vi "TreeItem.Get.vi"(6 "Custom Device Path":string, 8 "error in (no error)":errorcluster, 9 "Tree":T1[](array[typedef]) {"Properties"."Type" items=["K_STRING", "K_BOOL", "K_I32", "K_U32", "K_DOUBLE", "K_U64", "K_VARIANT", "K_DEPENDENTFILE", "K_DEPENDENTNODE", "K_DATASOURCENODE", "K_U16", "K_DBLARR", "K_U32ARR", "K_I32ARR", "K_STRINGARR", "K_DICTIONARY", "K_DICTIONARYARR"]}, 10 "BaseNode Ref":refnum<k24>, 11 "NodeIDUtil Ref":refnum<k24>) -> (0 "error out":errorcluster, 1 "Tree":T1[](array[typedef]) {"Properties"."Type" items=["K_STRING", "K_BOOL", "K_I32", "K_U32", "K_DOUBLE", "K_U64", "K_VARIANT", "K_DEPENDENTFILE", "K_DEPENDENTNODE", "K_DATASOURCENODE", "K_U16", "K_DBLARR", "K_U32ARR", "K_I32ARR", "K_STRINGARR", "K_DICTIONARY", "K_DICTIONARYARR"]}, 2 "BaseNode Ref out":refnum<k24>, 3 "NodeIDUtil Ref out":refnum<k24>)   [LabVIEW 2016, in "Advanced System Definition.lvlib"]
uses:
  SysDef API/Advanced System Definition.lvlib
  _Types/TreeItem.ctl
  _Types/TreeItem.Info.ctl
  <vilib>/NI Veristand/Custom Device API/Custom Device Channel.ctl
  <vilib>/NI Veristand/Custom Device API/Custom Device Channel Type.ctl
  <vilib>/NI Veristand/Custom Device API/Custom Device Waveform.ctl
  <vilib>/NI Veristand/Custom Device API/Custom Device Waveform DataType.ctl
  _Types/TreeItem.Property.ctl
  NationalInstruments.VeriStand.SystemStorage
  NationalInstruments.VeriStand.SystemDefinitionAPI
  <vilib>/NI VeriStand/Custom Device API/Custom Device API.lvlib
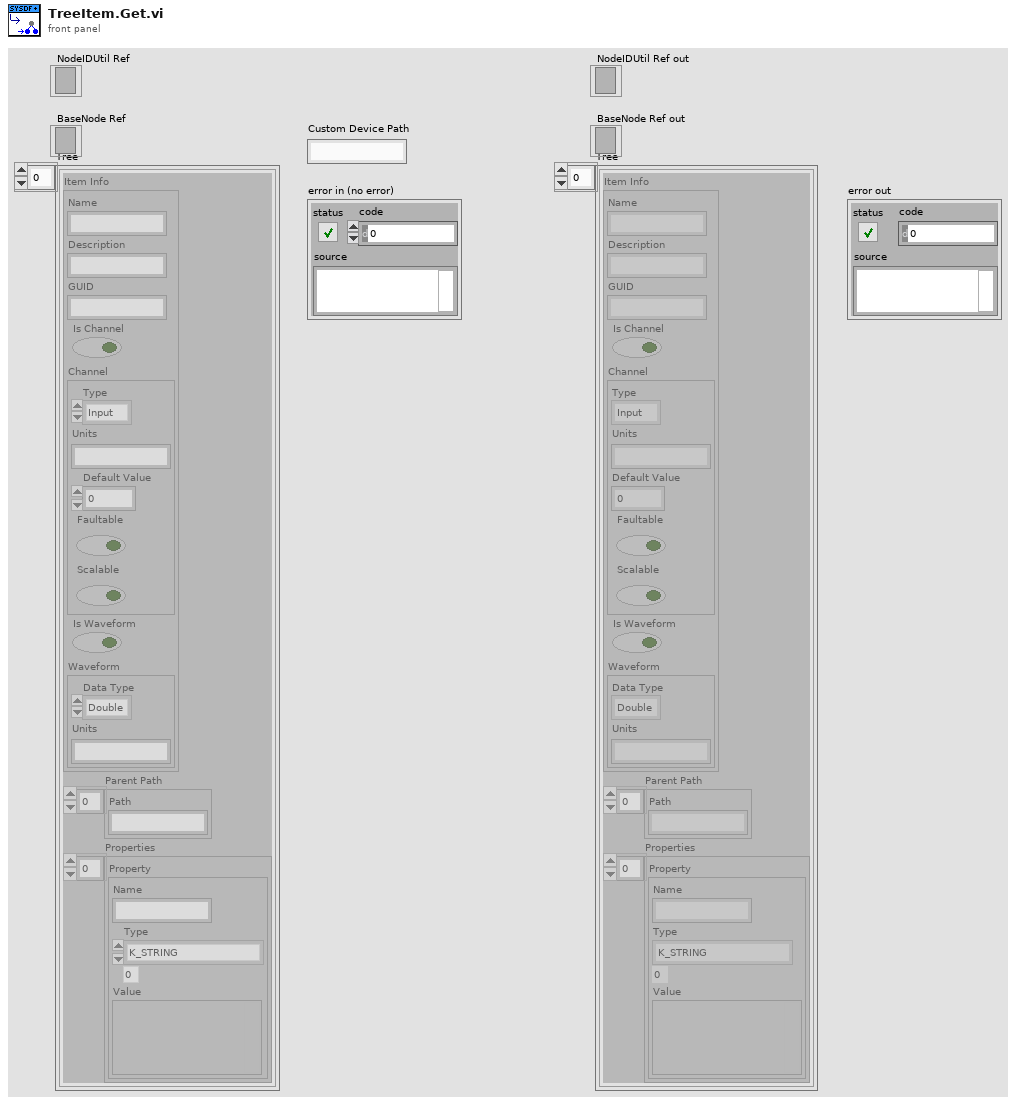
[diagram p1: front panel]
types:
  T1 = typedef "Advanced System Definition.lvlib/TreeItem.ctl" = cluster{"Item Info":T2, "Parent Path":string[], "Properties":T7[]}
  T2 = typedef "Advanced System Definition.lvlib/TreeItem.Info.ctl" = cluster{"Name":string, "Description":string, "GUID":string, "Is Channel":bool, "Channel":T3, "Is Waveform":bool, "Waveform":T5}
  T3 = typedef "Custom Device API.lvlib/Custom Device Channel.ctl" = cluster{"Type":T4, "Units":string, "Default Value":dbl, "Faultable":bool, "Scalable":bool}
  T4 = typedef "Custom Device API.lvlib/Custom Device Channel Type.ctl" = enum16{"Input", "Output"}
  T5 = typedef "Custom Device API.lvlib/Custom Device Waveform.ctl" = cluster{"Data Type":T6, "Units":string}
  T6 = typedef "Custom Device API.lvlib/Custom Device Waveform DataType.ctl" = enum16{"Double", "Complex Double"}
  T7 = typedef "Advanced System Definition.lvlib/TreeItem.Property.ctl" = cluster{"Name":string, "Type":i32, "Value":variant}
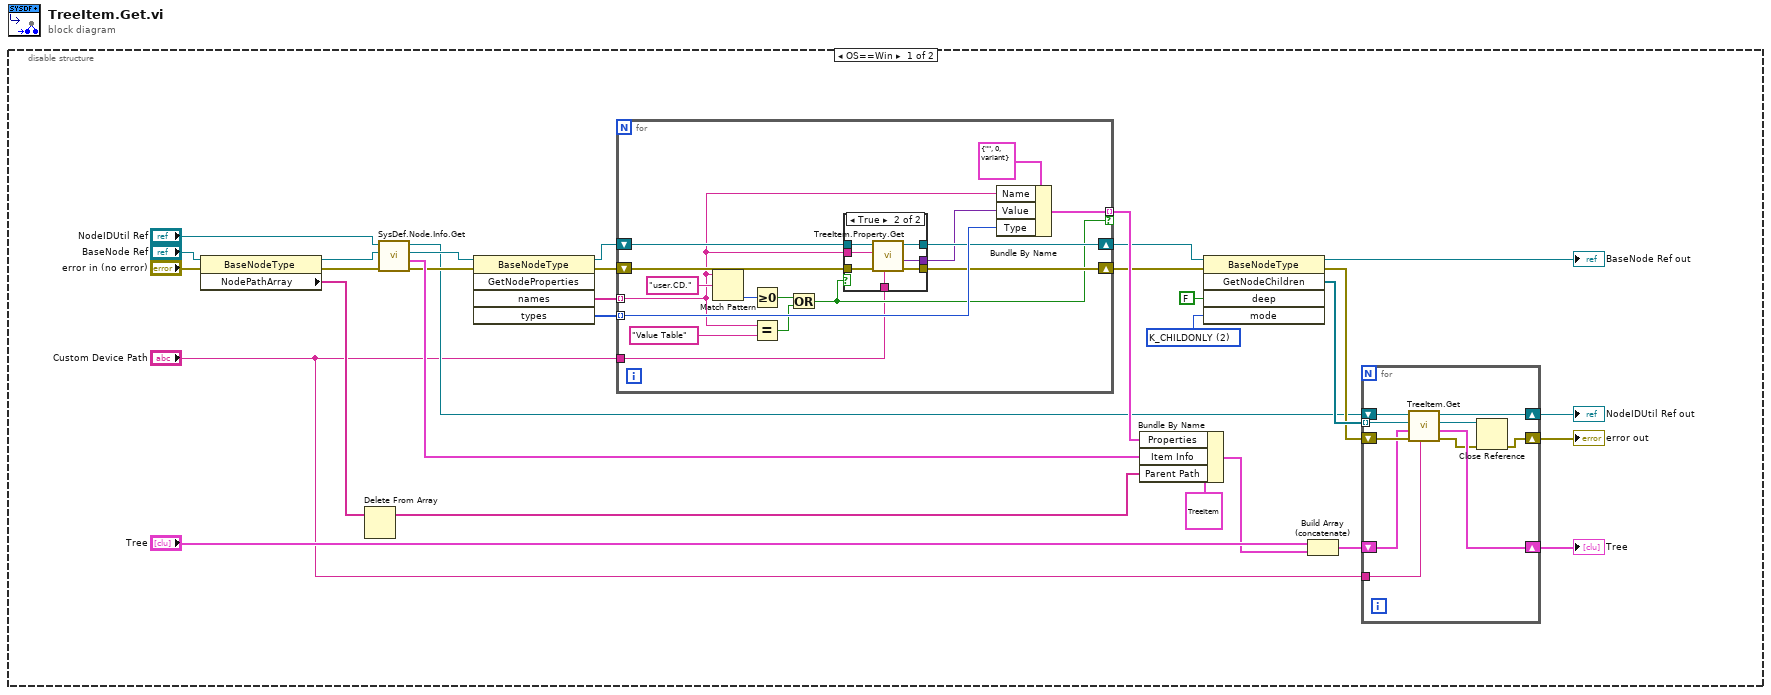
[diagram p0: block diagram]
diagram:
  n1 = disable-structure shown="OS==Win" {
    frame condition #0 (active) {
      w18 = 2 items=["K_BFS", "K_DFS", "K_CHILDONLY", "K_UP"] ("mode")
      n2 = property class="BaseNodeType"(reference="BaseNode Ref", error in="error in (no error)") -> (reference out=w6:refnum<k24>, error out=w9:errorcluster, "NodePathArray"=w7:string[])
      n3 = Delete From Array(array=w7) -> (array with subset deleted=w12:string[])  [unwired: 2 in, 1 out]
      n4 = call "SysDef.Node.Info.Get.vi"("error in (no error)"=w9, "BaseNode Ref"=w6, "NodeIDUtil Ref in"="NodeIDUtil Ref") -> ("error out"=w14:errorcluster, "Item Info"=w23:T2, "BaseNode Ref out"=w5:refnum<k24>, "NodeIDUtil Ref out"=w4:refnum<k24>)  [unwired: 5 in]
      n5 = invoke class="BaseNodeType" method="GetNodeProperties"(reference=w5, error in=w14) -> (reference out=w25:refnum<k24>, error out=w26:errorcluster, "names"=w28:string[], "types"=w27:i32[])  [unwired: 3 in, 1 out]
      n6 = for {
        tunnel: w27 -> [w52] mode=indexing
        tunnel: w28 -> [w47] mode=indexing
        shift-right: [w48] -> w21
        shift-left: w26 -> [w55]
        tunnel: [w51] -> w22 mode=indexing if=w43
        shift-right: [w50] -> w20
        shift-left: w25 -> [w54]
        tunnel: "Custom Device Path" -> [w42]
        n7 = Match Pattern(string=w47, regular expression="user.CD.") -> (offset past match=w56:i32)  [unwired: 1 in, 3 out]
        n8 = Greater Or Equal To 0?(x=w56) -> (x >= 0?=w44:bool)
        n9 = Equal?(x=w47, y="Value Table") -> (x = y?=w45:bool)
        n10 = Or(x=w44, y=w45) -> (x .or. y?=w43:bool)
        n11 = case shown="True" w43 {
          tunnel: w55 -> [w59 w66]
          tunnel: [w59 w65] -> w48
          tunnel: [_ w64] -> w49
          tunnel: w54 -> [w58 w63]
          tunnel: w47 -> [_ w62]
          tunnel: [w58 w61] -> w50
          tunnel: w42 -> [_ w60]
          frame False {
          }
          frame True {
            n12 = call "TreeItem.Property.Get.vi"("Custom Device Path"=w60, "error in (no error)"=w66, "Property Name"=w62, "Basenode"=w63) -> ("error out"=w65:errorcluster, "Variant"=w64:variant, "Basenode"=w61:refnum<k24>)  [unwired: 4 in, 1 out]
          }
        }
        n13 = Bundle By Name(cluster=T7 {"Name"="", "Type"=0, "Value"=variant(string "")}, "Name"=w47, "Value"=w49, "Type"=w52) -> (w51:T7)
      }
      n14 = Bundle By Name(cluster=T1 {"Item Info"={"Name"="", "Description"="", "GUID"="", "Is Channel"=FALSE, "Channel"={"Type"=enum."Input", "Units"="", "Default Value"=0.0, "Faultable"=FALSE, "Scalable"=FALSE}, "Is Waveform"=FALSE, "Waveform"={"Data Type"=enum."Double", "Units"=""}}, "Parent Path"=[], "Properties"=[]}, "Properties"=w22, "Item Info"=w23, "Parent Path"=w12) -> (w17:T1)
      n15 = invoke class="BaseNodeType" method="GetNodeChildren"(reference=w20, error in=w21, "deep"=FALSE, "mode"=w18) -> (reference out=→"BaseNode Ref out":refnum<k24>, error out=w13:errorcluster, "GetNodeChildren"=w16:refnum<k24>[])  [unwired: 1 in, 2 out]
      n16 = Build Array (concatenate)("Tree", w17) -> (w15:T1[])
      n17 = for {
        tunnel: w16 -> [w38] mode=indexing
        shift-right: [w39] -> w31
        shift-left: w15 -> [w40]
        shift-right: [w34] -> w29
        shift-left: w13 -> [w41]
        shift-right: [w36] -> w11
        shift-left: w4 -> [w37]
        tunnel: "Custom Device Path" -> [w32]
        n18 = call "TreeItem.Get.vi"("Custom Device Path"=w32, "error in (no error)"=w41, "Tree"=w40, "BaseNode Ref"=w38, "NodeIDUtil Ref"=w37) -> ("error out"=w35:errorcluster, "Tree"=w39:T1[], "BaseNode Ref out"=w33:refnum<k24>, "NodeIDUtil Ref out"=w36:refnum<k24>)  [unwired: 3 in]
        n19 = Close Reference(reference=w33, error in (no error)=w35) -> (error out=w34:errorcluster)
      }
      "Tree" <- w31
      "error out" <- w29
      "NodeIDUtil Ref out" <- w11
    }
    frame condition #1 {
    }
  }
